vi "Get All Test Results (Extended).vi"(6 "Filter Orphaned Tests? (F)":bool, 8 "error in (no error)":errorcluster, 11 "Test Result in":refnum<class "Test Result.lvclass">) -> (0 "error out":errorcluster, 2 "Test Results":T1[](array[typedef]), 3 "Test Result out":refnum<class "Test Result.lvclass">)   [LabVIEW 2013, in "Caraya.lvlib" / "Test Result.lvclass"]
uses:
  Test Result.lvclass
  Node Results (Extended).ctl
  Test Node (Extended).ctl
  Test Registration Data.ctl
  Assert Event Data (Extended).ctl
  Test Result.lvclass/Test Result.ctl
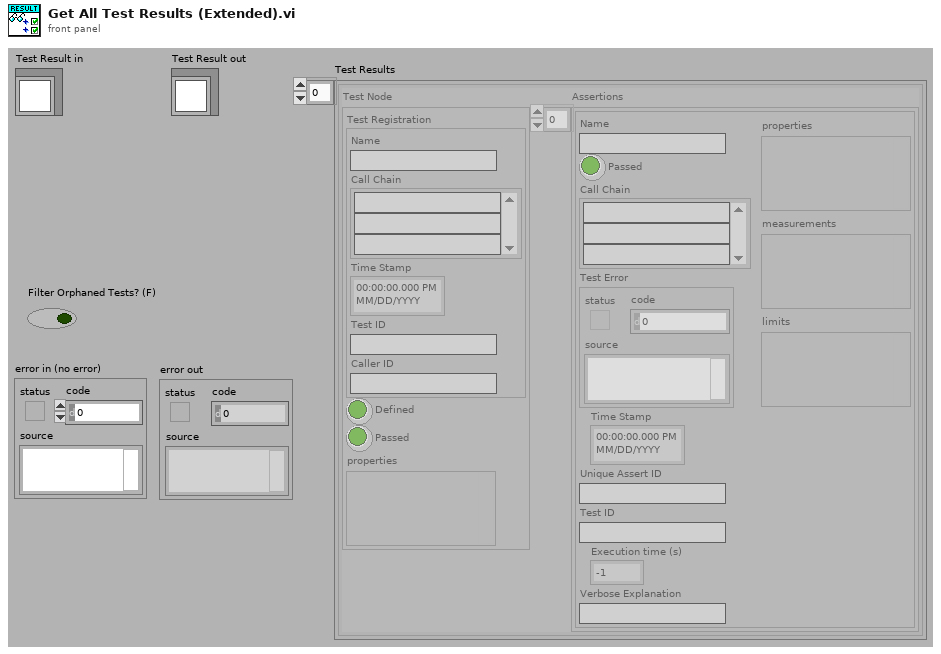
[diagram p1: front panel]
types:
  T1 = typedef "Caraya.lvlib/Test Result.lvclass/Node Results (Extended).ctl" = cluster{"Test Node":T2, "Assertions":T4[]}
  T2 = typedef "Caraya.lvlib/Test Result.lvclass/Test Node (Extended).ctl" = cluster{"Test Registration":T3, "Defined":bool, "Passed":bool, "properties":variant}
  T3 = typedef "Caraya.lvlib/Test Result.lvclass/Test Registration Data.ctl" = cluster{"Name":string, "Call Chain":string[], "Time Stamp":timestamp, "Test ID":string, "Caller ID":string}
  T4 = typedef "Caraya.lvlib/Test Result.lvclass/Assert Event Data (Extended).ctl" = cluster{"Name":string, "Passed":bool, "Call Chain":string[], "Test Error":errorcluster, "Time Stamp":timestamp, "Unique Assert ID":string, "Test ID":string, "Execution time (s)":dbl, "Verbose Explanation":string, "properties":variant, "measurements":variant, "limits":variant}
  T5 = cluster{i32, "Time Stamp":timestamp, "Caller ID":string, "Test ID":string, "Extended Node Result":T1}
  T6 = cluster{i32, "Time Stamp":timestamp, "Caller ID":string, "Test ID":string, "Extended Node Result":T1}[]
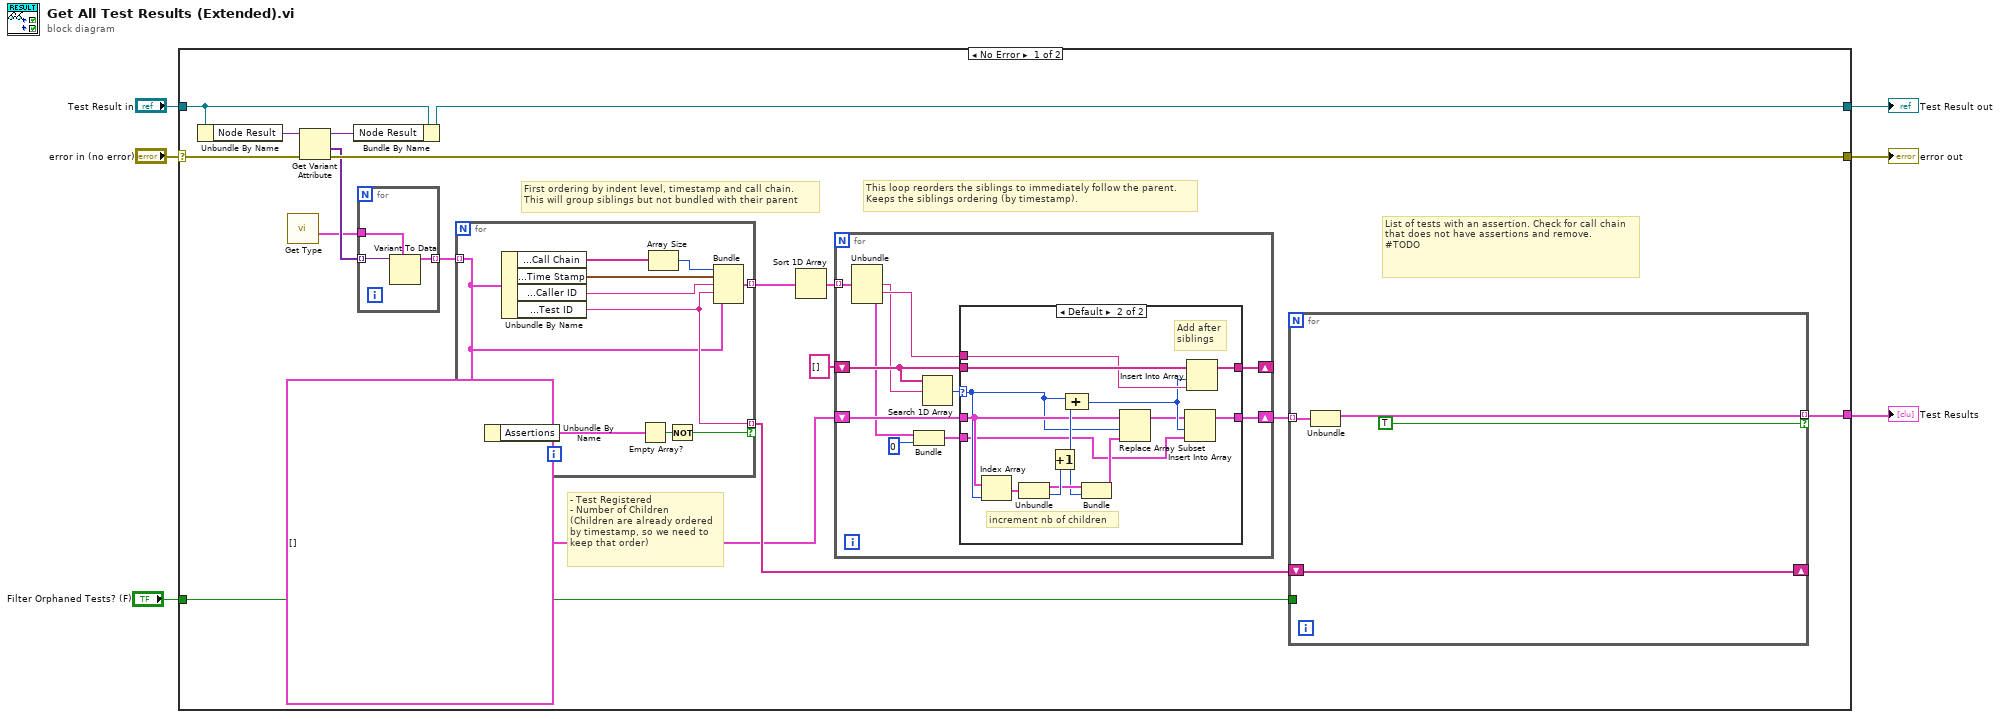
[diagram p0: block diagram]
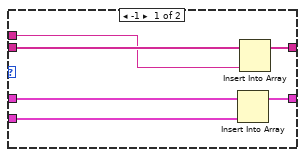
[diagram p2: hidden frame]
diagram:
  n1 = case shown="No Error" "error in (no error)" {
    selector: "error in (no error)" -> [w18 w73]
    tunnel: [w19 w73] -> w5
    tunnel: [w22 w72] -> w3
    tunnel: "Test Result in" -> [w23 w72]
    tunnel: [w11 _] -> w2
    tunnel: "Filter Orphaned Tests? (F)" -> [w9 _]
    frame No Error {
      # "List of tests with an assertion. Check for call chain that does not have assertions and remove.\n#TODO"
      # "First ordering by indent level, timestamp and call chain.\nThis will group siblings but not bundled with their parent"
      # "- Test Registered\n- Number of Children\n(Children are already ordered\nby timestamp, so we need to \nkeep that order)"
      # "This loop reorders the siblings to immediately follow the parent.\nKeeps the siblings ordering (by timestamp)."
      n2 = Unbundle By Name(w23) -> ("Node Result"=w21:variant)
      n3 = call "Get Type.vi"() -> ("Extended Node Result"=w8:T1)  [unwired: 10 in, 1 out]
      n4 = Get Variant Attribute(Variant=w21, error in=w18) -> (duplicate Variant=w20:variant, values=w17:variant[], error out=w19:errorcluster)  [unwired: 2 in, 1 out]
      n5 = Bundle By Name(cluster=w23, "Node Result"=w20) -> (w22:refnum<class "Test Result.lvclass">)
      n6 = for {
        tunnel: w17 -> [w71] mode=indexing
        tunnel: [w70] -> w16 mode=indexing
        tunnel: w8 -> [w69]
        n7 = Variant To Data(type=w69, Variant=w71) -> (data=w70:T1)  [unwired: 1 in, 1 out]
      }
      n8 = for {
        tunnel: w16 -> [w59] mode=indexing
        tunnel: [w68] -> w14 mode=indexing
        tunnel: [w61] -> w10 mode=indexing if=w63
        n9 = Unbundle By Name(w59) -> ("Assertions"=w60:T4[])
        n10 = Unbundle By Name(w59) -> ("Test Node.Test Registration.Call Chain"=w66:string[], "Test Node.Test Registration.Time Stamp"=w65:timestamp, "Test Node.Test Registration.Caller ID"=w62:string, "Test Node.Test Registration.Test ID"=w61:string)
        n11 = Empty Array?(array=w60) -> (empty?=w64:bool)
        n12 = Array Size(array=w66) -> (size(s)=w67:i32)
        n13 = Not(x=w64) -> (.not. x?=w63:bool)
        n14 = Bundle(w67, "Time Stamp"=w65, "Caller ID"=w62, "Test ID"=w61, "Extended Node Result"=w59) -> (w68:T5)  [unwired: 1 in]
      }
      n15 = Sort 1D Array(array=w14) -> (sorted array=w15:T6)
      n16 = for {
        tunnel: w15 -> [w38] mode=indexing
        shift-right: [w36] -> w12
        shift-left: cluster{"Node Result 2":T1, i32}[] [] -> [w37]
        shift-right: [w34] -> _
        shift-left: string[] [] -> [w33]
        n17 = Unbundle(w38) -> ("Caller ID"=w29:string, "Test ID"=w30:string, "Extended Node Result"=w28:T1)  [unwired: 2 out]
        n18 = Bundle("Extended Node Result"=w28, 0) -> (w31:cluster{"Extended Node Result":T1, i32})  [unwired: 1 in]
        n19 = Search 1D Array(1D array=w33, element=w29) -> (index of element=w35:i32)  [unwired: 1 in]
        n20 = case shown="Default" w35 {
          selector: w35 -> [_ w47]
          tunnel: w37 -> [w44 w49]
          tunnel: [w43 w58] -> w36
          tunnel: w31 -> [w42 w45]
          tunnel: w33 -> [w41 w57]
          tunnel: [w40 w56] -> w34
          tunnel: w30 -> [w39 w55]
          frame -1 {
            n21 = Insert Into Array(array=w44, new element=w42) -> (w43:cluster{"Node Result 2":T1, i32}[])  [unwired: 1 in]
            n22 = Insert Into Array(array=w41, new element=w39) -> (w40:string[])  [unwired: 1 in]
          }
          frame Default {
            # "Add after\nsiblings"
            # "increment nb of children"
            n23 = Index Array(array=w49, index=w47) -> (element=w54:cluster{"Node Result 2":T1, i32})
            n24 = Unbundle(w54) -> ("Node Result 2"=w51:T1, w53:i32)
            n25 = Increment(x=w53) -> (x+1=w50:i32)
            n26 = Compound Arithmetic op=ADD(w47, w50) -> (w52:i32)
            n27 = Bundle("Node Result 2"=w51, w50) -> (w46:cluster{"Node Result 2":T1, i32})  [unwired: 1 in]
            n28 = Replace Array Subset(array=w49, new element=w46, index=w47) -> (w48:cluster{"Node Result 2":T1, i32}[])
            n29 = Insert Into Array(array=w48, index=w52, new element=w45) -> (w58:cluster{"Node Result 2":T1, i32}[])
            n30 = Insert Into Array(array=w57, index=w52, new element=w55) -> (w56:string[])
          }
        }
      }
      n31 = for {
        tunnel: w12 -> [w27] mode=indexing
        tunnel: [w26] -> w11 mode=indexing if=TRUE
        tunnel: w9 -> [_]
        shift-right: [w24] -> _
        shift-left: w10 -> [w24]
        n32 = Unbundle(w27) -> ("Node Result 2"=w26:T1)  [unwired: 1 out]
      }
    }
    frame Error {
    }
  }
  "error out" <- w5
  "Test Result out" <- w3
  "Test Results" <- w2
